vi "DI SEQ Check.vi"() -> ()   [LabVIEW 2022 SP3]
uses:
  RT Sub VI's/RT Global.vi
panel:
  in  "DI read":bool[](array[boolean])=[FALSE, FALSE, FALSE, FALSE, FALSE, FALSE, FALSE]
  in  "DI":T1(array[cluster])=[{"CDT"=-150.0, "Position"=TRUE, "Component ID"="F_EPV_131", "Con(T)-Cum(F)"=FALSE, "No.of.Sam"=0.0, "Abort File"="", "Duration"=0}, {"CDT"=-150.0, "Position"=TRUE, "Component ID"="F_EPV_131", "Con(T)-Cum(F)"=FALSE, "No.of.Sam"=0.0, "Abort File"="", "Duration"=0}, {"CDT"=-135.0, "Position"=FALSE, "Component ID"="F_EPV_132", "Con(T)-Cum(F)"=FALSE, "No.of.Sam"=0.0, "Abort File"="", "Duration"=0}, {"CDT"=-120.0, "Position"=FALSE, "Component ID"="F_EPV_131", "Con(T)-Cum(F)"=FALSE, "No.of.Sam"=0.0, "Abort File"="", "Duration"=0}, {"CDT"=-20.0, "Position"=TRUE, "Component ID"="F_EPV_136", "Con(T)-Cum(F)"=FALSE, "No.of.Sam"=0.0, "Abort File"="", "Duration"=0}, {"CDT"=-10.0, "Position"=FALSE, "Component ID"="F_EPV_136", "Con(T)-Cum(F)"=FALSE, "No.of.Sam"=0.0, "Abort File"="", "Duration"=0}]
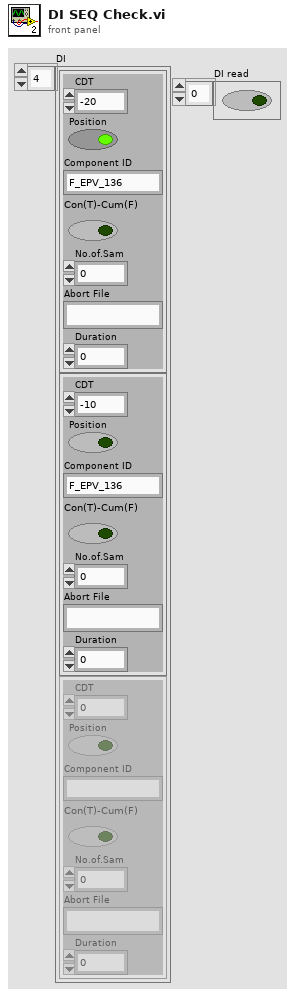
[diagram p1: front panel]
types:
  T1 = cluster{"CDT":dbl, "Position":bool, "Component ID":string, "Con(T)-Cum(F)":bool, "No.of.Sam":dbl, "Abort File":string, "Duration":u32}[]
  T2 = cluster{"AO":cluster{"CDT":dbl, "Range":dbl, "Component ID":string}[], "DO":cluster{"CDT":dbl, "Position":bool, "Component ID":string}[], "Launch Time":timestamp}
  T3 = cluster{"CDT":dbl, "Position":bool, "Component ID":string, "Con(T)-Cum(F)":bool, "No.of.Sam":dbl, "Abort File":string, "Duration":u32}
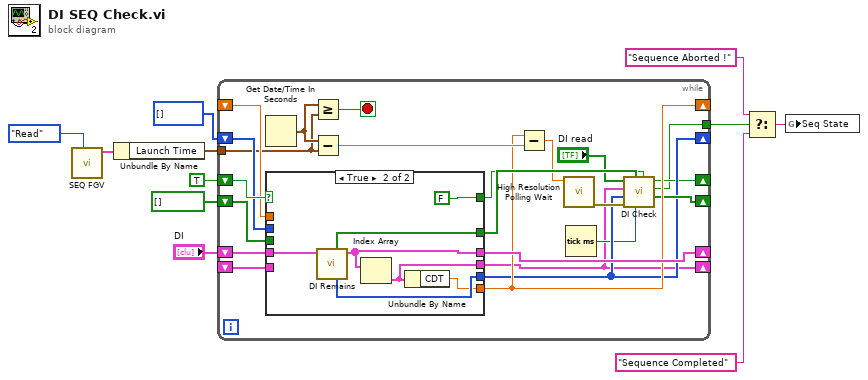
[diagram p0: block diagram]
diagram:
  n1 = call "SEQ FGV.vi"("Enum"=enum16{"Read", "Write"}."Read") -> ("Seq data out"=w9:T2)  [unwired: 9 in, 1 out]
  n2 = Unbundle By Name(w9) -> ("Launch Time"=w3:timestamp)
  n3 = while {
    shift-right: [w33] -> _
    shift-left: "DI" -> [w34]
    shift-right: [w20] -> _
    shift-left: bool[] [] ("DO value") -> [w30]
    shift-right: [w22] -> _
    shift-left: _ -> [w31]
    shift-right: [w17] -> _
    shift-left: TRUE -> [w32]
    shift-right: [w19] -> _
    shift-left: i32[] [] ("DI Index") -> [w29]
    tunnel: w3 -> [w27]
    tunnel: [w16] -> w1
    shift-right: [w14] -> _
    shift-left: _ -> [w13]
    stop <- w25 stop-if-true
    n4 = Get Date/Time In Seconds() -> (seconds since 1Jan1904=w28:timestamp)
    n5 = case shown="True" w32 {
      selector: w32 -> [w36 _]
      tunnel: w34 -> [w38 w42]
      tunnel: [w38 w45] -> w33
      tunnel: [w39 w47] -> w26
      tunnel: [w37 w46] -> w19
      tunnel: [w40 w44] -> w22
      tunnel: w31 -> [w40 _]
      tunnel: w30 -> [w39 _]
      tunnel: w29 -> [w37 _]
      tunnel: [w36 FALSE] -> w18
      tunnel: [w35 w41] -> w14
      tunnel: w13 -> [w35 _]
      frame False {
      }
      frame True {
        n6 = call "DI Remains.vi"("DI"=w42) -> ("Remains"=w45:T1, "DI Index"=w46:i32[], "DI value"=w47:bool[])  [unwired: 7 in, 1 out]
        n7 = Index Array(array=w45) -> (element=w41:T3)  [unwired: 1 in]
        n8 = Unbundle By Name(w41) -> ("CDT"=w44:dbl)
      }
    }
    n9 = Greater Or Equal?(x=w28, y=w27) -> (x >= y?=w25:bool)
    n10 = Subtract(x=w28, y=w27) -> (x-y=w23:dbl)
    n11 = Subtract(x=w22, y=w23) -> (x-y=w21:dbl)
    n12 = call <vilib>:"High Resolution Polling Wait.vi"("seconds to wait"=w21) -> ("error out"=w24:errorcluster)  [unwired: 10 in]
    n13 = Tick Count (ms)() -> (millisecond timer value=w15:u32)
    n14 = call "DI Check.vi"("Boolean in"=w18, "millisecond timer value"=w15, "DI value in"=w26, "error in (no error)"=w24, "DI Index"=w19, "Cluster"=w14, "DI read"="DI read") -> ("DI value out"=w20:bool[], "Abort Seq"=w16:bool, "Boolean out"=w17:bool)  [unwired: 2 in]
  }
  n15 = Select(t="Sequence Aborted !" ("Seq State"), s=w1, f="Sequence Completed" ("Seq State")) -> (s? t:f=w6:string)
  n16 = global write "RT Global.vi" "Seq State"(w6) -> ()
